vi "Servo.vi"() -> ()   [LabVIEW 2012]
uses:
  <vilib>/robotics/Utilities/FPGA Utilities/NI_Robotics_FPGA Utilities.lvlib
  <vilib>/robotics/Utilities/FPGA Utilities/Generate Digital Pulse (uSec).vi
  <instrlib>/Hitec HS400 Series/FPGA/NI_Robotics_Hitec HS400 Series (FPGA).lvlib
panel:
  in  "Servo":T1={"Period (us)"=20000, "Pulse width (us)"=15000}
  in  "Servo":refnum<k21>="DIO0"
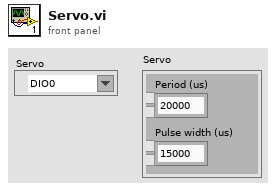
[diagram p1: front panel]
types:
  T1 = cluster{"Period (us)":u32, "Pulse width (us)":u32}
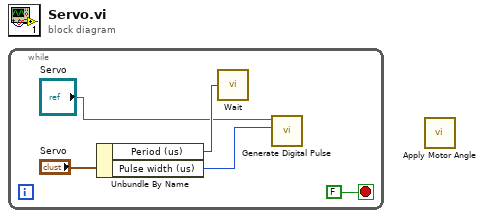
[diagram p0: block diagram]
diagram:
  n1 = while {
    stop <- FALSE stop-if-true
    n2 = Unbundle By Name("Servo") -> ("Period (us)"=w3:u32, "Pulse width (us)"=w4:u32)
    n3 = call "Wait"("Count(uSec)"=w3) -> ()  [unwired: 1 out]
    n4 = call-poly <vilib>:"Generate Digital Pulse.vi"("pulse width (uSec)"=w4, "FPGA digital output"="Servo") -> ()  [unwired: 10 in]
  }
  n5 = call <instrlib>:"Apply Motor Angle.vi"() -> ()  [unwired: 12 in]
